vi "GateDelay_Control_V1.vi"() -> ()   [LabVIEW 2014]
uses:
  GateDelayAction_TypeDef.ctl
  <vilib>/Utility/file.llb/Write To Spreadsheet File (DBL).vi
panel:
  in  "GO":bool
  in  "5":bool
  in  "4":bool
  in  "3":bool
  in  "2":bool
  in  "1":bool
  in  "0":bool
  in  "Exit":bool
  in  "Window Width (ns)":dbl(slide) min=0.0 max=9.7904 step=0.0095703125 scale=0.0..10.0
  in  "Window Delay (ns)":dbl(slide) min=0.0 max=19.9902 step=0.009765625 scale=0.0..20.0
  in  "Laser Delay (ns)":dbl(slide) min=0.0 max=19.9902 step=0.009765625 scale=0.0..20.0
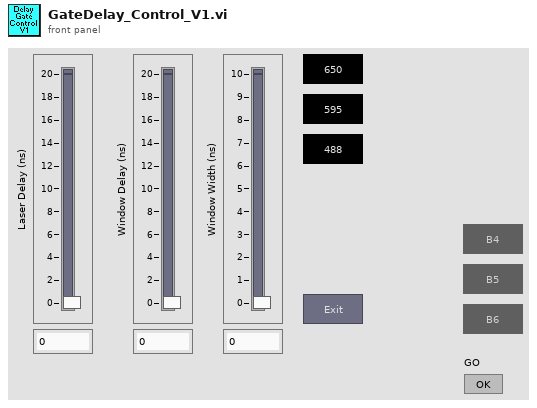
[diagram p1: front panel]
types:
  T1 = typedef "GateDelayAction_TypeDef.ctl" = enum16{"Set Laser Delay", "Set Window Delay", "Set Window Width", "Get Delays", "Exit", "CloseConnections", "Initialize"}
  T2 = enum8{"Enabled", "Disabled", "Disabled and Grayed Out"}
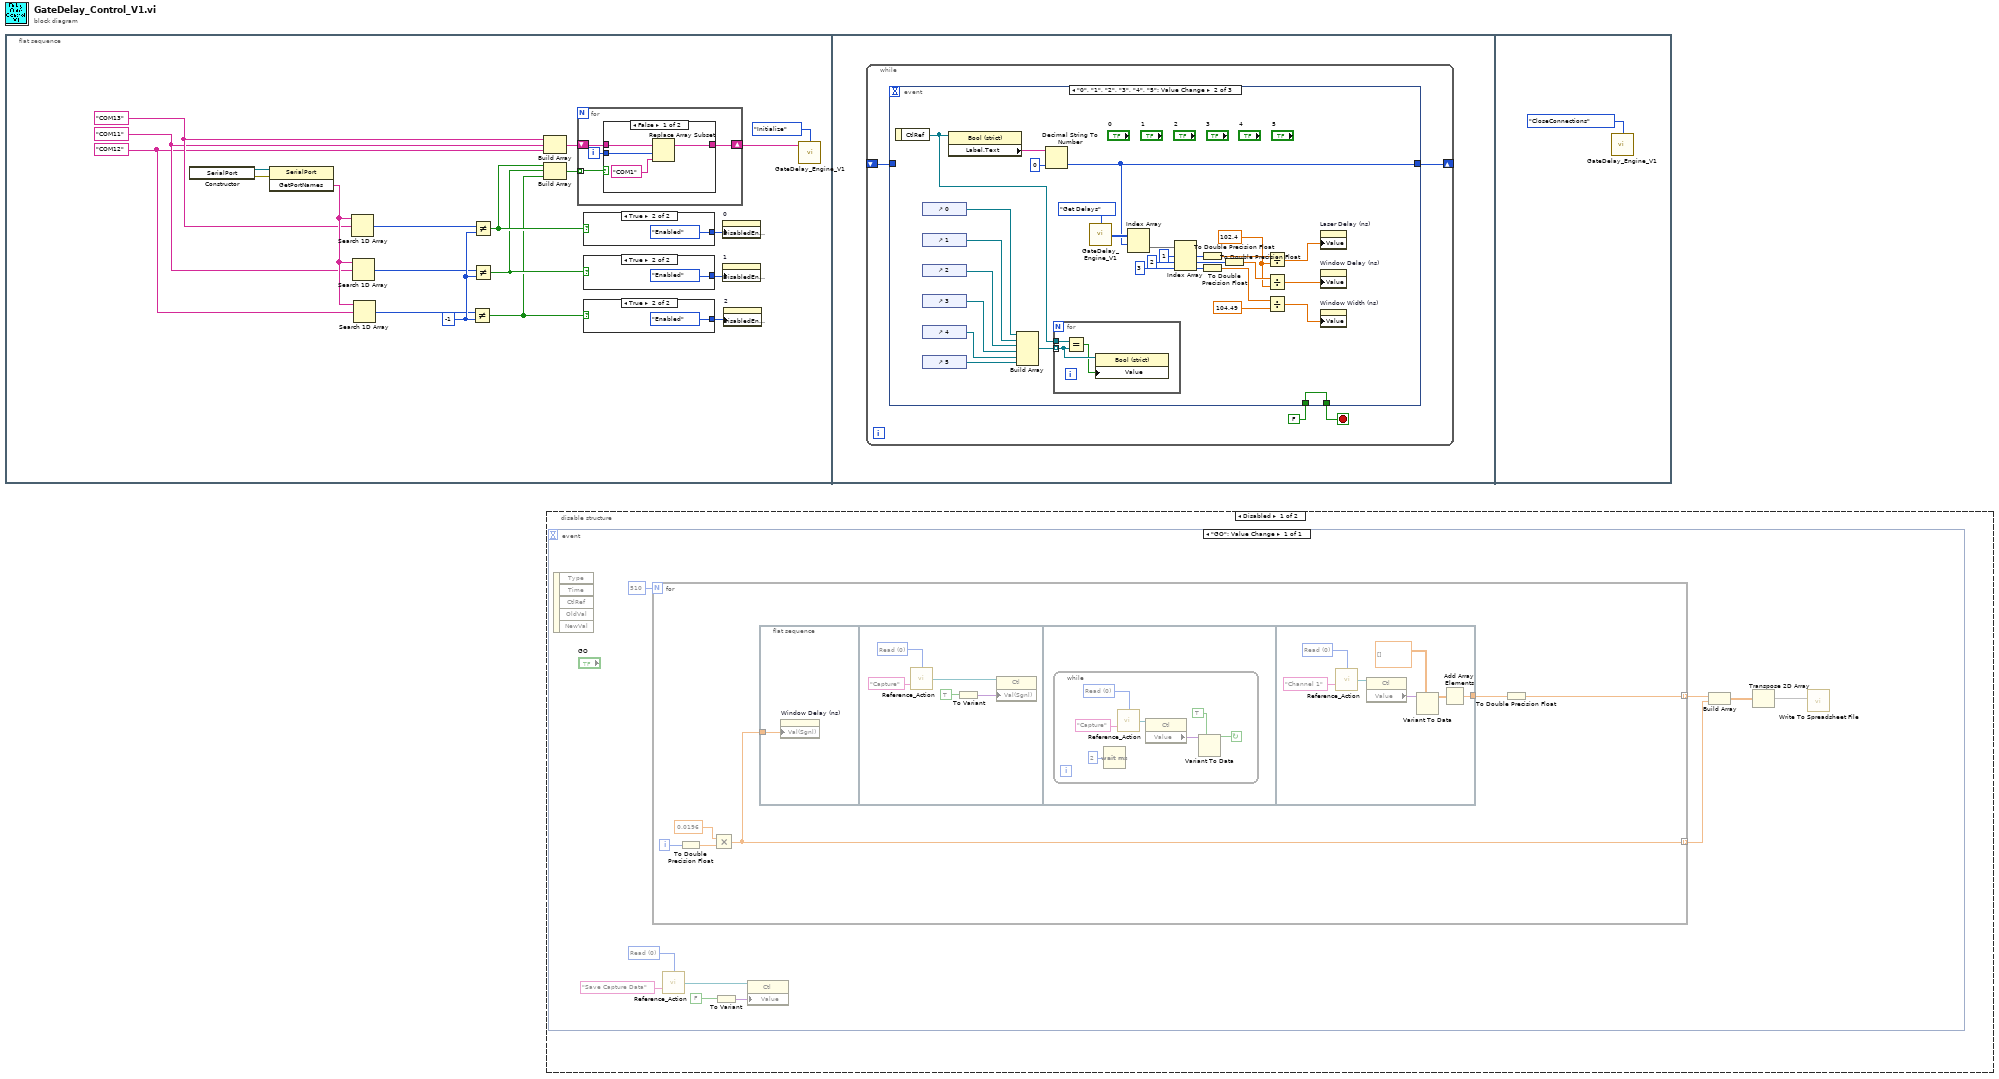
[diagram p0: block diagram]
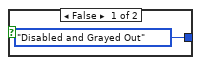
[diagram p4: hidden frame]
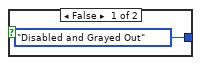
[diagram p5: hidden frame]
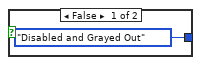
[diagram p6: hidden frame]
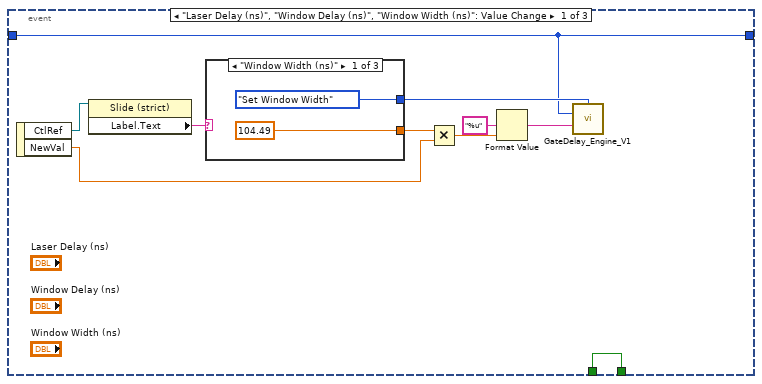
[diagram p7: hidden frame]
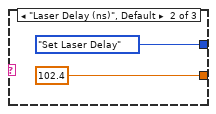
[diagram p8: hidden frame]
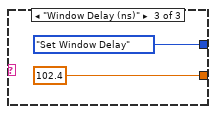
[diagram p9: hidden frame]
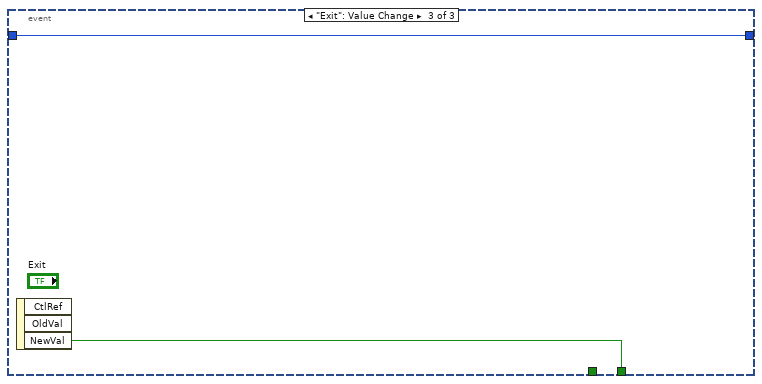
[diagram p10: hidden frame]
diagram:
  n1 = flat-sequence {
    frame #0 {
      w10 = -1 ("y")
      w1 = "COM12"
      w2 = "COM11"
      w3 = "COM13"
      n2 = constructor class="SerialPort"() -> (reference out=w9:refnum<k24>, error out=w8:errorcluster)  [unwired: 3 in, 1 out]
      n3 = invoke class="SerialPort" method="GetPortNames"(reference=w9, error in=w8) -> ("GetPortNames"=w5:string[])  [unwired: 1 in, 2 out]
      n4 = Search 1D Array(1D array=w5, element=w3) -> (index of element=w7:i32)  [unwired: 1 in]
      n5 = Search 1D Array(1D array=w5, element=w2) -> (index of element=w6:i32)  [unwired: 1 in]
      n6 = Search 1D Array(1D array=w5, element=w1) -> (index of element=w4:i32)  [unwired: 1 in]
      n7 = Not Equal?(x=w4, y=w10) -> (x != y?=w14:bool)
      n8 = Not Equal?(x=w7, y=w10) -> (x != y?=w16:bool)
      n9 = Not Equal?(x=w6, y=w10) -> (x != y?=w15:bool)
      n10 = Build Array(w3, w2, w1) -> (w12:string[])
      n11 = Build Array(w16, w15, w14) -> (w13:bool[])
      n12 = for {
        tunnel: w13 -> [w24] mode=indexing
        shift-right: [w21] -> w11
        shift-left: w12 -> [w23]
        i -> [w22]
        n13 = case shown="False" w24 {
          tunnel: w23 -> [w28 w29]
          tunnel: w22 -> [w27 _]
          tunnel: [w26 w29] -> w21
          frame False {
            n14 = Replace Array Subset(array=w28, new element="COM1" ("new element/subarray"), index=w27) -> (w26:string[])
          }
          frame True {
          }
        }
      }
      n15 = case shown="True" w16 {
        tunnel: [T2."Disabled and Grayed Out" ("Disabled") T2."Enabled" ("Disabled")] -> w19
        frame False {
        }
        frame True {
        }
      }
      n16 = case shown="True" w15 {
        tunnel: [T2."Disabled and Grayed Out" ("Disabled") T2."Enabled" ("Disabled")] -> w18
        frame False {
        }
        frame True {
        }
      }
      n17 = case shown="True" w14 {
        tunnel: [T2."Disabled and Grayed Out" ("Disabled") T2."Enabled" ("Disabled")] -> w17
        frame False {
        }
        frame True {
        }
      }
      n18 = property on="0" class="Bool (strict)"("DisabledEnum"=w19) -> ()  [unwired: 2 in, 2 out]
      n19 = property on="1" class="Bool (strict)"("DisabledEnum"=w18) -> ()  [unwired: 2 in, 2 out]
      n20 = property on="2" class="Bool (strict)"("DisabledEnum"=w17) -> ()  [unwired: 2 in, 2 out]
      n21 = call "GateDelay_Engine_V1.vi"("Port Array"=w11, "DelayGate Action"=GateDelayAction_TypeDef."Initialize") -> ()  [unwired: 13 in, 1 out]
    }
    frame #1 {
      n22 = while {
        shift-right: [w37] -> _
        shift-left: _ -> [w36]
        stop <- w39 stop-if-true
        n23 = event shown="[1] \"0\", \"1\", \"2\", \"3\", \"4\", \"5\": Value Change" {
          selector: _ -> [_ _ _]
          dyn-events: _ -> [_ _ _]
          timeout: _ -> [_ _ _]
          tunnel: [w41 w84 w89] -> w39
          tunnel: FALSE -> [w41 w84 _]
          tunnel: [w40 w71 w88] -> w37
          tunnel: w36 -> [w40 _ w88]
          event "Laser Delay (ns)", "Window Delay (ns)", "Window Width (ns)": Value Change {
            n24 = event-data() -> ("CtlRef"=w49:refnum<vi>, "NewVal"=w46:dbl)  [unwired: 1 in]
            n25 = property class="Slide (strict)"(reference=w49) -> ("Label.Text"=w48:string)  [unwired: 1 in, 2 out]
            n26 = case shown="\"Window Width (ns)\"" w48 {
              tunnel: [GateDelayAction_TypeDef."Set Window Width" ("DelayGate Action") GateDelayAction_TypeDef."Set Laser Delay" ("DelayGate Action") GateDelayAction_TypeDef."Set Window Delay" ("DelayGate Action")] -> w42
              tunnel: [104.49 102.4 102.4] -> w47
              frame "Window Width (ns)" {
              }
              frame "Laser Delay (ns)", Default {
              }
              frame "Window Delay (ns)" {
              }
            }
            n27 = Multiply(x=w47, y=w46) -> (x*y=w45:dbl)
            n28 = Format Value(format string="%u", value (0)=w45) -> (output string=w43:string)  [unwired: 1 in]
            n29 = call "GateDelay_Engine_V1.vi"("DelayGate Action"=w42, "Device Index"=w40, "Delay Value (steps)"=w43) -> ()  [unwired: 12 in, 1 out]
          }
          event "0", "1", "2", "3", "4", "5": Value Change {
            w59 = 102.4
            n30 = event-data() -> ("CtlRef"=w74:refnum<vi>)  [unwired: 1 in]
            n31 = control-ref of="0"() -> (w81:refnum<vi>)
            n32 = control-ref of="1"() -> (w80:refnum<vi>)
            n33 = control-ref of="2"() -> (w79:refnum<vi>)
            n34 = control-ref of="3"() -> (w78:refnum<vi>)
            n35 = control-ref of="4"() -> (w77:refnum<vi>)
            n36 = control-ref of="5"() -> (w76:refnum<vi>)
            n37 = property class="Bool (strict)"(reference=w74) -> ("Label.Text"=w83:string)  [unwired: 1 in, 2 out]
            n38 = Build Array(w81, w80, w79, w78, w77, w76) -> (w75:refnum<vi>[])
            n39 = Decimal String To Number(string=w83, default (0L)=0 ("default (0 I32)")) -> (number=w71:i32)  [unwired: 1 in, 1 out]
            n40 = for {
              tunnel: w75 -> [w86] mode=indexing
              tunnel: w74 -> [w87]
              n41 = Equal?(x=w87, y=w86) -> (x = y?=w85:bool)
              n42 = property class="Bool (strict)"(reference=w86, "Value"=w85) -> ()  [unwired: 1 in, 2 out]
            }
            n43 = call "GateDelay_Engine_V1.vi"("DelayGate Action"=GateDelayAction_TypeDef."Get Delays") -> ("Current Delays"=w72:i32[][])  [unwired: 14 in]
            n44 = Index Array(array=w72, index (row)=w71) -> (element=w70:i32[])  [unwired: 1 in]
            n45 = Index Array(array=w70, index #1=1 ("index"), index #2=2 ("index"), index #3=3 ("index")) -> (element #1=w66:i32, element #2=w65:i32, element #3=w64:i32)
            n46 = To Double Precision Float(number=w66) -> (double precision float=w63:dbl)
            n47 = To Double Precision Float(number=w64) -> (double precision float=w61:dbl)
            n48 = To Double Precision Float(number=w65) -> (double precision float=w62:dbl)
            n49 = Divide(x=w63, y=w59) -> (x/y=w56:dbl)
            n50 = Divide(x=w62, y=w59) -> (x/y=w58:dbl)
            n51 = Divide(x=w61, y=104.49) -> (x/y=w57:dbl)
            n52 = property on="Laser Delay (ns)" class="Slide (strict)"("Value"=w56) -> ()  [unwired: 2 in, 2 out]
            n53 = property on="Window Delay (ns)" class="Slide (strict)"("Value"=w58) -> ()  [unwired: 2 in, 2 out]
            n54 = property on="Window Width (ns)" class="Slide (strict)"("Value"=w57) -> ()  [unwired: 2 in, 2 out]
          }
          event "Exit": Value Change {
            n55 = event-data() -> ("NewVal"=w89:bool)  [unwired: 1 in, 2 out]
          }
        }
      }
    }
    frame #2 {
      n56 = call "GateDelay_Engine_V1.vi"("DelayGate Action"=GateDelayAction_TypeDef."CloseConnections") -> ()  [unwired: 14 in, 1 out]
    }
  }
  n57 = disable-structure shown="Disabled" {
    frame Disabled {
      n58 = event shown="[0] \"GO\": Value Change" {
        selector: _ -> [_]
        dyn-events: _ -> [_]
        timeout: _ -> [_]
        event "GO": Value Change {
          w96 = u16 0 items=["Read", "Initialize"] ("Action")
          n59 = event-data() -> ()  [unwired: 1 in, 5 out]
          n60 = for {
            N: 510 -> [_]
            tunnel: [w103] -> w93 mode=indexing
            tunnel: [w101] -> w94 mode=indexing
            i -> [w106]
            n61 = To Double Precision Float(number=w106) -> (double precision float=w105:dbl)
            n62 = Multiply(x=0.0196, y=w105) -> (x*y=w103:dbl)
            n63 = flat-sequence {
              tunnel: w103 -> [w107]
              tunnel: [w120] -> w102
              frame #0 {
                n64 = property on="Window Delay (ns)" class="Slide (strict)"("Val(Sgnl)"=w107) -> ()  [unwired: 2 in, 2 out]
              }
              frame #1 {
                w112 = u16 0 items=["Read", "Initialize"] ("Action")
                n65 = call "Reference_Action.vi"("Action"=w112, "Control Name"="Capture") -> ("Ref OUT"=w110:refnum<vi>)  [unwired: 12 in, 1 out]
                n66 = To Variant(anything=TRUE) -> (Variant=w108:variant)
                n67 = property class="Ctl"(reference=w110, "Val(Sgnl)"=w108) -> ()  [unwired: 1 in, 2 out]
              }
              frame #2 {
                n68 = while {
                  stop <- w114 continue-if-true
                  w117 = u16 0 items=["Read", "Initialize"] ("Action")
                  n69 = Wait (ms)(milliseconds to wait=u32 2) -> ()  [unwired: 1 out]
                  n70 = call "Reference_Action.vi"("Action"=w117, "Control Name"="Capture") -> ("Ref OUT"=w119:refnum<vi>)  [unwired: 12 in, 1 out]
                  n71 = property class="Ctl"(reference=w119) -> ("Value"=w116:variant)  [unwired: 1 in, 2 out]
                  n72 = Variant To Data(type=TRUE, Variant=w116) -> (data=w114:bool)  [unwired: 1 in, 1 out]
                }
              }
              frame #3 {
                w125 = u16 0 items=["Read", "Initialize"] ("Action")
                n73 = call "Reference_Action.vi"("Action"=w125, "Control Name"="Channel 1") -> ("Ref OUT"=w124:refnum<vi>)  [unwired: 12 in, 1 out]
                n74 = property class="Ctl"(reference=w124) -> ("Value"=w123:variant)  [unwired: 1 in, 2 out]
                n75 = Variant To Data(type=sgl[][] [], Variant=w123) -> (data=w121:sgl[][])  [unwired: 1 in, 1 out]
                n76 = Add Array Elements(numeric array=w121) -> (sum=w120:sgl)
              }
            }
            n77 = To Double Precision Float(number=w102) -> (double precision float=w101:dbl)
          }
          n78 = call "Reference_Action.vi"("Action"=w96, "Control Name"="Save Capture Data") -> ("Ref OUT"=w97:refnum<vi>)  [unwired: 12 in, 1 out]
          n79 = To Variant(anything=FALSE) -> (Variant=w98:variant)
          n80 = property class="Ctl"(reference=w97, "Value"=w98) -> ()  [unwired: 1 in, 2 out]
          n81 = Build Array(w94, w93) -> (w92:dbl[][])
          n82 = Transpose 2D Array(2D array=w92) -> (transposed array=w91:dbl[][])
          n83 = call-poly <vilib>:"Write To Spreadsheet File.vi"("2D data"=w91) -> ()  [unwired: 7 in, 1 out]
        }
      }
    }
    frame Enabled {
    }
  }
